vi "SetBinning.vi"(6 "SupportedBinning":refnum<k24>, 7 "Y Binning":refnum<vi>, 9 "Settings":refnum<k24>, 10 "X Binning":refnum<vi>, 11 "ComboBox in":refnum<vi>) -> ()   [LabVIEW 2019]
uses:
  Dependencies/PVCamNET.dll
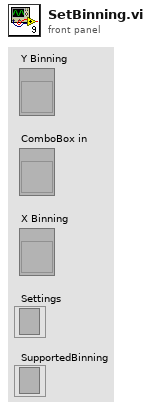
[diagram p1: front panel]
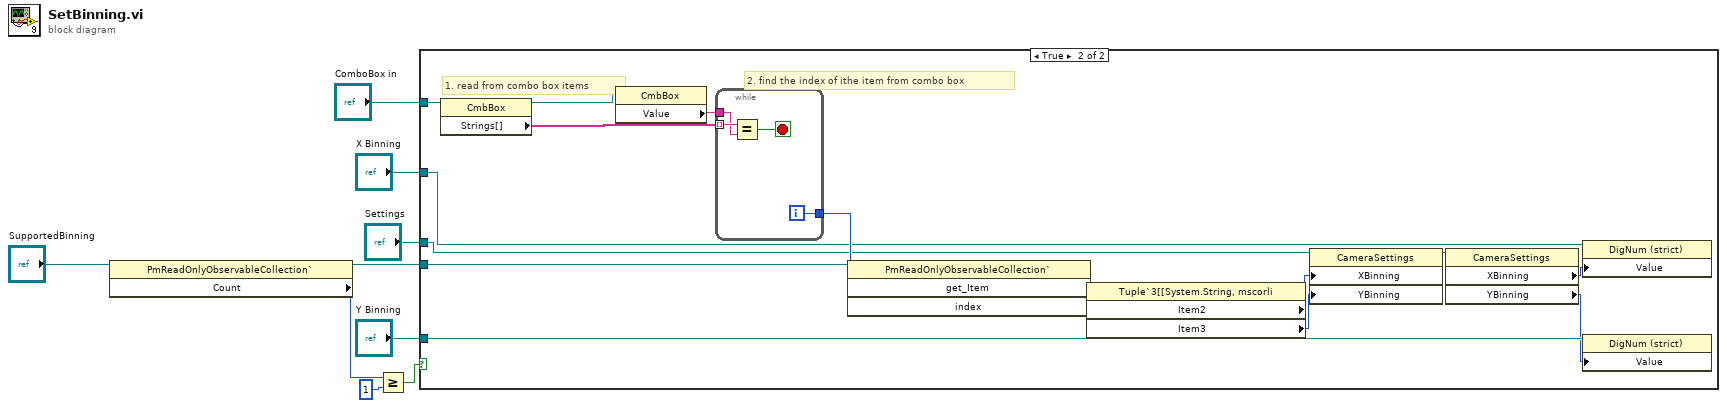
[diagram p0: block diagram]
diagram:
  n1 = property class="PmReadOnlyObservableCollection`"(reference="SupportedBinning") -> (reference out=w5:refnum<k24>, "Count"=w4:i32)  [unwired: 1 in, 1 out]
  n2 = Greater Or Equal?(x=w4, y=u16 1) -> (x >= y?=w6:bool)
  n3 = case shown="True" w6 {
    tunnel: "Settings" -> [_ w18]
    tunnel: w5 -> [_ w17]
    tunnel: "ComboBox in" -> [_ w16]
    tunnel: "X Binning" -> [_ w13]
    tunnel: "Y Binning" -> [_ w12]
    frame False {
    }
    frame True {
      # "2. find the index of ithe item from combo box"
      # "1. read from combo box items"
      n4 = property class="CmbBox"(reference=w16) -> (reference out=w15:refnum<vi>, "Strings[]"=w24:string[])  [unwired: 1 in, 1 out]
      n5 = property class="CmbBox"(reference=w15) -> ("Value"=w14:string)  [unwired: 1 in, 2 out]
      n6 = while {
        tunnel: w24 -> [w28] mode=indexing
        tunnel: [w26] -> w23
        tunnel: w14 -> [w25]
        i -> [w26]
        stop <- w27 stop-if-true
        n7 = Equal?(x=w28, y=w25) -> (x = y?=w27:bool)
      }
      n8 = invoke class="PmReadOnlyObservableCollection`" method="get_Item"(reference=w17, "index"=w23) -> ("get_Item"=w22:refnum<k24>)  [unwired: 2 in, 3 out]
      n9 = property class="Tuple`3[[System.String, mscorli"(reference=w22) -> ("Item2"=w21:u16, "Item3"=w20:u16)  [unwired: 1 in, 2 out]
      n10 = property class="CameraSettings"(reference=w18, "XBinning"=w21, "YBinning"=w20) -> (reference out=w19:refnum<k24>)  [unwired: 1 in, 1 out]
      n11 = property class="CameraSettings"(reference=w19) -> ("XBinning"=w10:u16, "YBinning"=w11:u16)  [unwired: 1 in, 2 out]
      n12 = property class="DigNum (strict)"(reference=w13, "Value"=w10) -> ()  [unwired: 1 in, 2 out]
      n13 = property class="DigNum (strict)"(reference=w12, "Value"=w11) -> ()  [unwired: 1 in, 2 out]
    }
  }
